vi "availableCodecs.vi"(8 "Error In":errorcluster) -> (0 "Error Out":errorcluster, 2 "Value":string[](array[string]))   [LabVIEW 2014, in "QTextCodec.lvclass"]
doc: "LabVIEW-specific documentation is not yet available. See <b>https://doc.qt.io/qt-5/qtextcodec.html#availableCodecs</b>"
uses:
  QTextCodec.lvclass
  LQ Core.lvlib
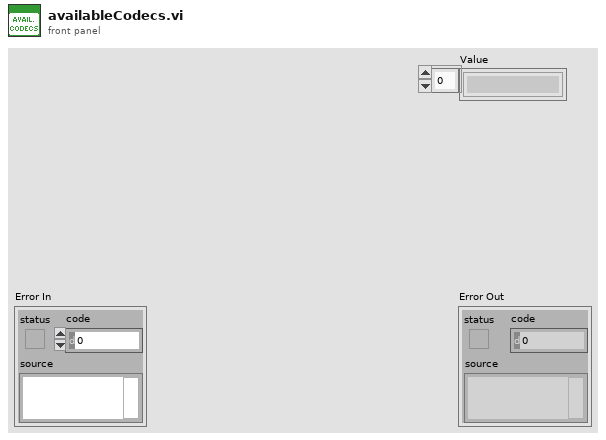
[diagram p1: front panel]
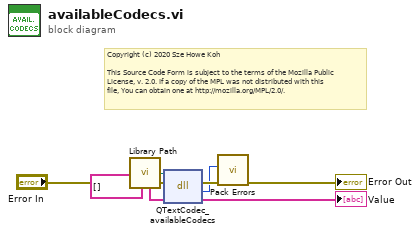
[diagram p0: block diagram]
diagram:
  # "Copyright (c) 2020 Sze Howe Koh\n\nThis Source Code Form is subject to the terms of the Mozilla Public\nLicense, v. 2.0. If a copy of the MPL was not distributed with this\nfile, You can obtain one at http://mozilla.org/MPL/2.0/."
  n1 = call "Library Path.vi"() -> ("Library Path"=w5:path)
  n2 = dll-call lib="?" fn="QTextCodec_availableCodecs"(path in=w5, error in="Error In", "_retVal"=string[] [] ("retVal")) -> (error out=w3:errorcluster, w1:i32, "_retVal"=→"Value":string[])  [unwired: 1 in, 1 out]
  n3 = call "Pack Errors.vi"("Error In"=w3, "Error Code"=w1) -> ("Error Out"=→"Error Out":errorcluster)  [unwired: 9 in]
